vi "TP - Read actual position.vi"(8 "error in":errorcluster, 10 "Axis":i8=1 min=1 max=6 step=1, 11 "Address / Port":i16=1 min=1 max=31 step=1) -> (0 "error out":errorcluster, 1 "Query the current actual\nposition - read":dbl, 2 "Axis dup":i8=1 min=1 max=6 step=1, 3 "Address / Port dup":i16=1 min=1 max=31 step=1)   [LabVIEW 2014]
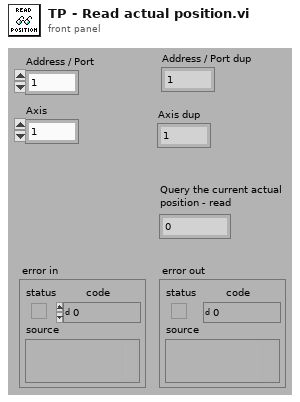
[diagram p1: front panel]
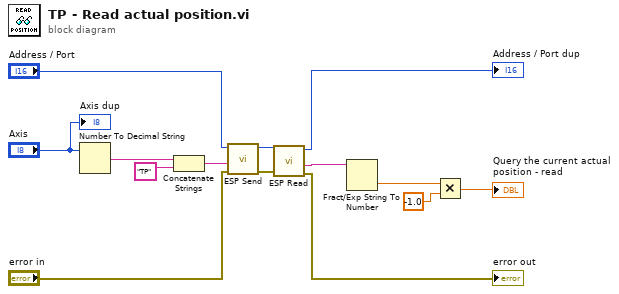
[diagram p0: block diagram]
diagram:
  n1 = Number To Decimal String(number="Axis") -> (decimal integer string=w13:string)  [unwired: 1 in]
  n2 = Concatenate Strings(w13, "TP" ("Substring")) -> (w11:string)
  n3 = call "ESP Send.vi"("error in"="error in", "Command String"=w11, "Address / Port"="Address / Port") -> ("error out"=w7:errorcluster, "Address / Port dup"=w6:i16)  [unwired: 3 in]
  n4 = call "ESP Read.vi"("error in"=w7, "Address / Port"=w6) -> ("error out"=→"error out":errorcluster, "Response String"=w4:string, "Address / Port dup"=→"Address / Port dup":i16)  [unwired: 3 in]
  n5 = Fract/Exp String To Number(string=w4) -> (number=w2:dbl)  [unwired: 3 in, 1 out]
  n6 = Multiply(x=w2, y=-1.0) -> (x*y=→"Query the current actual\nposition - read":dbl)
  "Axis dup" <- "Axis"
